vi "Digital Read.vi"   [LabVIEW 2014, in "LMH-LINX.lvlib"]
doc: "Read the value of the specified digital input channel(s)."
uses:
  <vilib>/MakerHub/LINX/LMH-LINX.lvlib
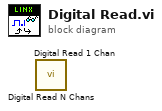
[diagram p0: block diagram]
diagram:
  n1 = call <vilib>:"Digital Read N Chans.vi"() -> ()  [unwired: 9 in, 3 out]
  n2 = call <vilib>:"Digital Read 1 Chan.vi"() -> ()  [unwired: 9 in, 3 out]
